vi "Umgebung.KalenderUhr.vi"(8 "Error in":errorcluster, 11 "Umgebung in":refnum<data-value>) -> (0 "Error out":errorcluster, 3 "Umgebung out":refnum<data-value>)   [LabVIEW 2016, in "Umgebung.lvclass"]
uses:
  Umgebung.lvclass
  Umgebung.lvclass/Umgebung.ctl
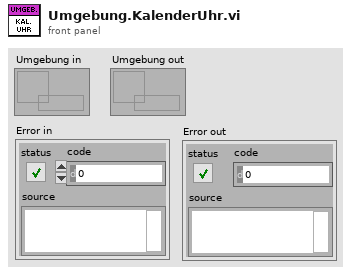
[diagram p1: front panel]
types:
  T1 = typedef "LVDateTimeRec.ctl" = cluster{"fractional second":dbl, "second":i32, "minute":i32, "hour":i32, "day of month":i32, "month":i32, "year":i32, "day of week":i32, "day of year":i32, "DST":i32}
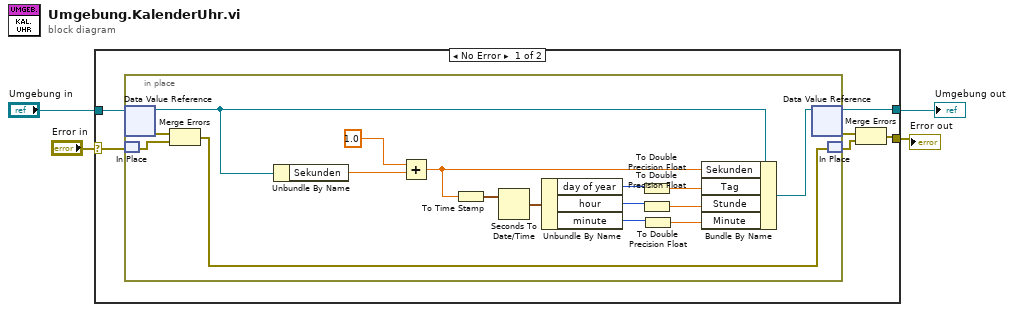
[diagram p0: block diagram]
diagram:
  n1 = case shown="No Error" "Error in" {
    selector: "Error in" -> [w7 w28]
    tunnel: [w8 w28] -> w1
    tunnel: [w10 w27] -> w3
    tunnel: "Umgebung in" -> [w5 w27]
    frame No Error {
      n2 = in-place {
        n3 = in-place-dvr #1(w5) -> (w23:refnum<class "Umgebung.lvclass">, w25:errorcluster)
        n4 = in-place-match #2(w7) -> (w24:errorcluster)
        n5 = Merge Errors(w25, w24) -> (w26:errorcluster)
        n6 = Unbundle By Name(w23) -> ("Sekunden"=w13:dbl)
        n7 = Add(x=1.0, y=w13) -> (x+y=w11:dbl)
        n8 = To Time Stamp(1:w11) -> (0:w12:timestamp)
        n9 = Seconds To Date/Time(time stamp (now)=w12) -> (date time rec=w20:T1)  [unwired: 1 in]
        n10 = Unbundle By Name(w20) -> ("day of year"=w19:i32, "hour"=w17:i32, "minute"=w15:i32)
        n11 = To Double Precision Float(number=w19) -> (double precision float=w18:dbl)
        n12 = To Double Precision Float(number=w17) -> (double precision float=w16:dbl)
        n13 = To Double Precision Float(number=w15) -> (double precision float=w14:dbl)
        n14 = Bundle By Name(cluster=w23, "Sekunden"=w11, "Tag"=w18, "Stunde"=w16, "Minute"=w14) -> (w22:refnum<class "Umgebung.lvclass">)
        n15 = in-place-dvr #1(w22) -> (w10:refnum<data-value>, w9:errorcluster)
        n16 = in-place-match #2(w26) -> (w6:errorcluster)
      }
      n17 = Merge Errors(w9, w6) -> (w8:errorcluster)
    }
    frame Error {
    }
  }
  "Umgebung out" <- w3
  "Error out" <- w1
